vi "QWTB Algorithms Filter Get List.vi"(11 "info data":string) -> (2 "algs list":string[](array[string]), 3 "info data out":string)   [LabVIEW 2020]
uses:
  octave/infolib/infolib.lvlib
  octave/infolib/Get 1D String.vi
  octave/infolib/GetString.vi
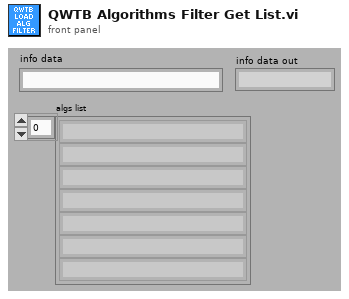
[diagram p1: front panel]
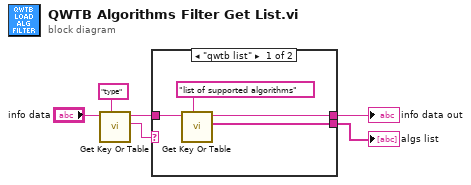
[diagram p0: block diagram]
diagram:
  n1 = call-poly "Get Key Or Table.vi"("key description"="type", "info data"="info data") -> ("value"=w3:string, "info data out"=w6:string)  [unwired: 6 in, 2 out]
  n2 = case shown="\"qwtb list\"" w3 {
    tunnel: w6 -> [w10 w11]
    tunnel: [w8 _] -> w2
    tunnel: [w7 w11] -> w1
    frame "qwtb list" {
      n3 = call-poly "Get Key Or Table.vi"("key description"="list of supported algorithms", "info data"=w10) -> ("value"=w8:string[], "info data out"=w7:string)  [unwired: 6 in, 2 out]
    }
    frame Default {
    }
  }
  "algs list" <- w2
  "info data out" <- w1
